vi "StopControl.vi"(8 "Reset":bool, 9 "Rate (unit/s)":dbl=0.5, 11 "Motor Value":dbl step=0.1) -> (0 "Done Stopping":bool, 3 "New Motor Value":dbl)   [LabVIEW 2012]
doc: "Stops a given motor value based on time since last call and given rate. Rate of change is always linear with respect to time. Designed to be run multiple times in while loop. Use shift register to maintain Motor Value in external while loop."
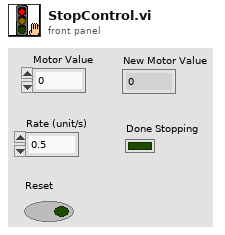
[diagram p1: front panel]
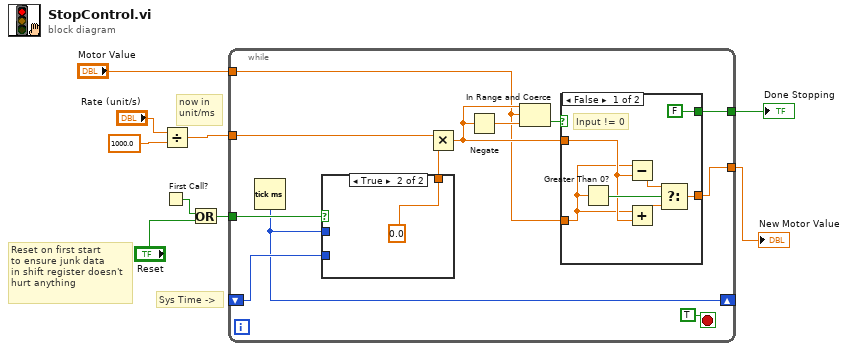
[diagram p0: block diagram]
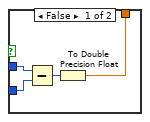
[diagram p2: hidden frame]
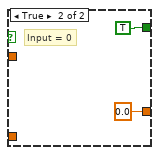
[diagram p3: hidden frame]
diagram:
  # "Sys Time ->"
  # "now in\nunit/ms"
  # "Reset on first start\nto ensure junk data\nin shift register doesn't\nhurt anything"
  n1 = First Call?() -> (First Call?: T/F=w5:bool)
  n2 = Divide(x="Rate (unit/s)", y=1000.0) -> (x/y=w6:dbl)
  n3 = Or(x=w5, y="Reset") -> (x .or. y?=w3:bool)
  n4 = while {
    tunnel: w6 -> [w19]
    tunnel: [w21] -> w9
    tunnel: w3 -> [w13]
    shift-right: [w11] -> _
    shift-left: _ -> [w12]
    tunnel: "Motor Value" -> [w16]
    tunnel: [w14] -> w1
    stop <- TRUE stop-if-true
    n5 = Tick Count (ms)() -> (millisecond timer value=w11:u32)
    n6 = case shown="True" w13 {
      tunnel: w12 -> [w24 _]
      tunnel: w11 -> [w25 _]
      tunnel: [w22 0.0] -> w10
      frame False {
        n7 = Subtract(x=w25, y=w24) -> (x-y=w23:u32)
        n8 = To Double Precision Float(number=w23) -> (double precision float=w22:dbl)
      }
      frame True {
      }
    }
    n9 = Multiply(x=w19, y=w10) -> (x*y=w17:dbl)
    n10 = Negate(x=w17) -> (-x=w18:dbl)
    n11 = In Range and Coerce(upper limit=w17, x=w16, lower limit=w18) -> (In Range?=w15:bool)  [unwired: 1 out]
    n12 = case shown="False" w15 {
      tunnel: [w30 0.0] -> w14
      tunnel: w17 -> [w28 _]
      tunnel: w16 -> [w27 _]
      tunnel: [FALSE TRUE] -> w21
      frame False {
        # "Input != 0"
        n13 = Greater Than 0?(x=w27) -> (x > 0?=w32:bool)
        n14 = Subtract(x=w27, y=w28) -> (x-y=w31:dbl)
        n15 = Add(x=w27, y=w28) -> (x+y=w29:dbl)
        n16 = Select(t=w31, s=w32, f=w29) -> (s? t:f=w30:dbl)
      }
      frame True {
        # "Input = 0"
      }
    }
  }
  "Done Stopping" <- w9
  "New Motor Value" <- w1
